vi "niFPGA BFGroup Twiddle Table 16 U64 Inv.vi"(7 "address":fxp<+,4,4>) -> (4 "twid real":fxp<+/-,33,2> format="%.32g", 6 "twid imag":fxp<+/-,33,2> format="%.32g")   [LabVIEW 2017]
uses:
  <vilib>/rvi/FXPMathLib/basic elements/FxpDiscreteDelay/XNode/nifxpmath_DiscreteDelay.xnode
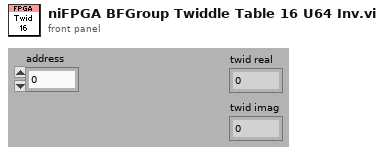
[diagram p1: front panel]
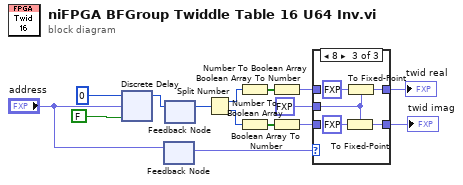
[diagram p0: block diagram]
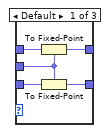
[diagram p2: hidden frame]
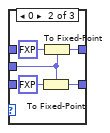
[diagram p3: hidden frame]
diagram:
  n1 = xnode "Discrete Delay"("D"=u64 0, "n-1[0..15]"="address", "enable"=FALSE) -> ("Q"=w8:u64)
  n2 = feedback-in #1("address") -> ()
  n3 = feedback #1() -> (w5:fxp<+,4,4>)  [unwired: 1 out]
  n4 = feedback-in #2(w8) -> ()
  n5 = feedback #2() -> (w11:u64)  [unwired: 1 out]
  n6 = Split Number(x=w11) -> (hi(x)=w14:u32, lo(x)=w12:u32)
  n7 = Number To Boolean Array(number=w14) -> (Boolean array=w15:bool[])
  n8 = Number To Boolean Array(number=w12) -> (Boolean array=w13:bool[])
  n9 = Boolean Array To Number(Boolean array=w15) -> (number=w7:fxp<+/-,32,1>)
  n10 = Boolean Array To Number(Boolean array=w13) -> (number=w6:fxp<+/-,32,1>)
  n11 = case shown="8" w5 {
    tunnel: w7 -> [w20 _ _]
    tunnel: [w19 w25 w30] -> w3
    tunnel: [w18 w22 w27] -> w2
    tunnel: w6 -> [w17 _ _]
    tunnel: fxp<+/-,33,2> 0.0 ("fixed-point type") -> [w16 w21 w26]
    frame Default {
      n12 = To Fixed-Point(fixed-point type=w16, number=w20) -> (fixed-point=w19:fxp<+/-,33,2>)
      n13 = To Fixed-Point(fixed-point type=w16, number=w17) -> (fixed-point=w18:fxp<+/-,33,2>)
    }
    frame 0 {
      n14 = To Fixed-Point(fixed-point type=w21, number=fxp<+,1,1> 0.0 ("fixed-point type")) -> (fixed-point=w22:fxp<+/-,33,2>)
      n15 = To Fixed-Point(fixed-point type=w21, number=fxp<+,1,1> 1.0 ("fixed-point type")) -> (fixed-point=w25:fxp<+/-,33,2>)
    }
    frame 8 {
      n16 = To Fixed-Point(fixed-point type=w26, number=fxp<+,1,1> 1.0 ("fixed-point type")) -> (fixed-point=w27:fxp<+/-,33,2>)
      n17 = To Fixed-Point(fixed-point type=w26, number=fxp<+,1,1> 0.0 ("fixed-point type")) -> (fixed-point=w30:fxp<+/-,33,2>)
    }
  }
  "twid real" <- w3
  "twid imag" <- w2
